vi "CheckForExistingErrorDialog.vi"(9 "ErrorIn":errorcluster, 11 "ErrorCodeIn":i32) -> (1 "ErrorOut":errorcluster, 2 "NoWndwFnd":bool, 3 "ErrorCodeOut":i32)   [LabVIEW 2018]
uses:
  <vilib>/Utility/sysdir.llb/System Directory Type.ctl
panel:
  out "Window Handle":i32
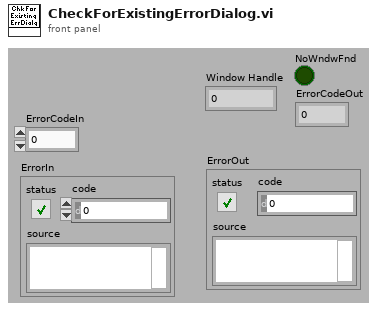
[diagram p1: front panel]
types:
  T1 = typedef "System Directory Type.ctl" = i32
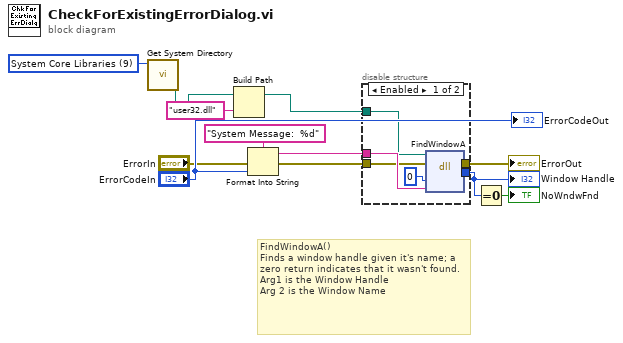
[diagram p0: block diagram]
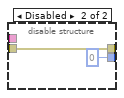
[diagram p2: hidden frame]
diagram:
  w4 = T1 9 items=["User Home"=0, "User Desktop"=1, "User Documents"=2, "User Application Data"=3, "User Preferences"=4, "User Temporary"=5, "Public Documents"=6, "Public Application Data"=7, "Public Preferences"=8, "Public Cache"=13, "System Core Libraries"=9, "System Installed Libraries"=10, "Application Files"=11, "Boot Volume Root"=12] ("system directory type")
  # "FindWindowA()\nFinds a window handle given it's name; a zero return indicates that it wasn't found.\nArg1 is the Window Handle\nArg 2 is the Window Name"
  n1 = call <vilib>:"Get System Directory.vi"("system directory type"=w4) -> ("system directory"=w3:path)  [unwired: 10 in]
  n2 = Build Path(base path=w3, name or relative path="user32.dll") -> (appended path=w2:path)
  n3 = Format Into String(format string="System Message:  %d" ("string"), error in="ErrorIn", "ErrorCodeIn") -> (resulting string=w7:string, error out=w5:errorcluster)  [unwired: 1 in]
  n4 = disable-structure shown="Enabled" {
    disable-tunnel: [w17 w20] -> w12
    disable-tunnel: [w16 0 ("Window Handle")] -> w11
    disable-tunnel: w7 -> [w15 _]
    disable-tunnel: w5 -> [w14 w20]
    disable-tunnel: w2 -> [w13 _]
    frame Enabled {
      n5 = dll-call lib="user32.dll" fn="FindWindowA"(path in=w13, error in=w14, "arg1"=0, "arg2"=w15) -> (error out=w17:errorcluster, "return type"=w16:i32)  [unwired: 2 in, 2 out]
    }
    frame Disabled {
    }
  }
  "Window Handle" <- w11
  "ErrorOut" <- w12
  n6 = Equal To 0?(x=w11) -> (x = 0?=→"NoWndwFnd":bool)
  "ErrorCodeOut" <- "ErrorCodeIn"
